vi "ScanivalveInit.vi"(0 "Scanner IP Address":string, 1 "Sampling Frequency Requested (Hz)":dbl, 2 "Total # of Samples to Collect":i32) -> (3 "TCP Network Connection out":refnum<k5>, 6 "error out":errorcluster)   [LabVIEW 2019]
panel:
  out "Sampling Frequency Set (Hz)":dbl=10.0 format="%#_6f"
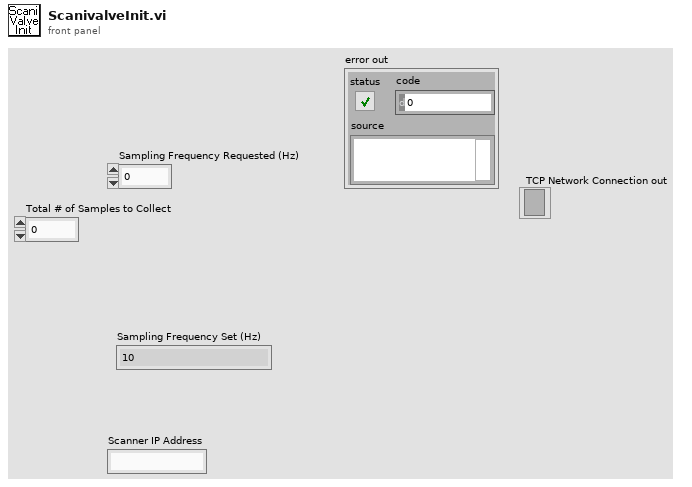
[diagram p1: front panel]
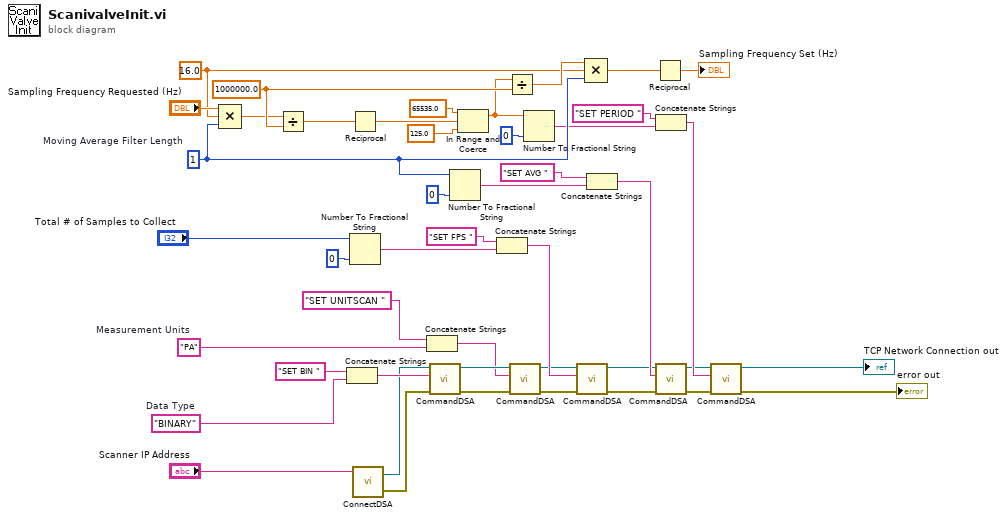
[diagram p0: block diagram]
diagram:
  w37 = i8 1  # Moving Average Filter Length
  w16 = "PA"  # Measurement Units
  w45 = "BINARY"  # Data Type
  w35 = 1000000.0 ("y")
  w31 = 16.0 ("x")
  n1 = Compound Arithmetic op=MULTIPLY("Sampling Frequency Requested (Hz)", w31, w37) -> (w28:dbl)
  n2 = Divide(x=w28, y=w35) -> (x/y=w33:dbl)
  n3 = Concatenate Strings("SET BIN ", w45) -> (w44:string)
  n4 = Reciprocal(x=w33) -> (1/x=w27:dbl)
  n5 = Number To Fractional String(number="Total # of Samples to Collect", precision (6)=i16 0) -> (F-format string=w7:string)  [unwired: 2 in]
  n6 = call "ConnectDSA.vi"("address"="Scanner IP Address") -> ("error out"=w39:errorcluster, "connection ID out"=w41:refnum<k5>)  [unwired: 3 in]
  n7 = Concatenate Strings("SET UNITSCAN ", w16) -> (w15:string)
  n8 = call "CommandDSA.vi"("error in (no error)"=w39, "command"=w44, "connection ID"=w41) -> ("error out"=w40:errorcluster, "connection ID out"=w42:refnum<k5>)  [unwired: 1 in, 2 out]
  n9 = Number To Fractional String(number=w37, precision (6)=i16 0) -> (F-format string=w19:string)  [unwired: 2 in]
  n10 = In Range and Coerce(upper limit=65535.0, x=w27, lower limit=125.0) -> (coerced(x)=w32:dbl)  [unwired: 1 out]
  n11 = Concatenate Strings("SET FPS ", w7) -> (w9:string)
  n12 = Divide(x=w32, y=w35) -> (x/y=w34:dbl)
  n13 = call "CommandDSA.vi"("error in (no error)"=w40, "command"=w15, "connection ID"=w42) -> ("error out"=w2:errorcluster, "connection ID out"=w1:refnum<k5>)  [unwired: 1 in, 2 out]
  n14 = Number To Fractional String(number=w32, precision (6)=i16 0) -> (F-format string=w23:string)  [unwired: 2 in]
  n15 = call "CommandDSA.vi"("error in (no error)"=w2, "command"=w9, "connection ID"=w1) -> ("error out"=w3:errorcluster, "connection ID out"=w4:refnum<k5>)  [unwired: 1 in, 2 out]
  n16 = Compound Arithmetic op=MULTIPLY(w34, w31, w37) -> (w30:dbl)
  n17 = Concatenate Strings("SET AVG ", w19) -> (w21:string)
  n18 = Reciprocal(x=w30) -> (1/x=→"Sampling Frequency Set (Hz)":dbl)
  n19 = Concatenate Strings("SET PERIOD ", w23) -> (w38:string)
  n20 = call "CommandDSA.vi"("error in (no error)"=w3, "command"=w21, "connection ID"=w4) -> ("error out"=w14:errorcluster, "connection ID out"=w13:refnum<k5>)  [unwired: 1 in, 2 out]
  n21 = call "CommandDSA.vi"("error in (no error)"=w14, "command"=w38, "connection ID"=w13) -> ("error out"=→"error out":errorcluster, "connection ID out"=→"TCP Network Connection out":refnum<k5>)  [unwired: 1 in, 2 out]
